vi "Koheras_AOTF.vi"(10 "String":string, 11 "VISA resource name 2":refnum<visa-resource-name>) -> (0 "error out":errorcluster, 2 "read buffer":string)   [LabVIEW 2009]
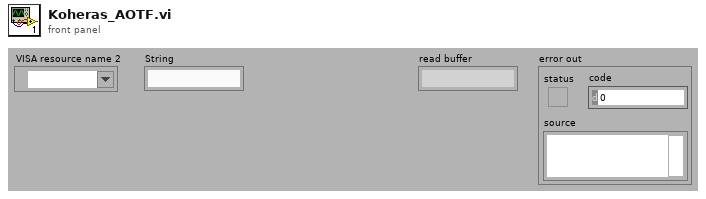
[diagram p1: front panel]
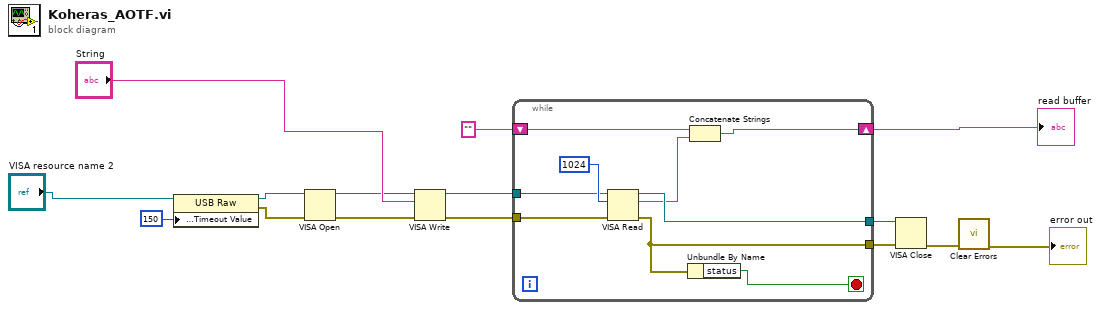
[diagram p0: block diagram]
diagram:
  n1 = property class="USB Raw"(reference="VISA resource name 2", "General Settings:Timeout Value"=u32 150) -> (reference out=w3:refnum<visa-resource-name>, error out=w2:errorcluster)  [unwired: 1 in]
  n2 = VISA Open(error in (no error)=w2, VISA resource name=w3) -> (VISA resource name=w8:refnum<visa-resource-name>, error out=w7:errorcluster)  [unwired: 3 out]
  n3 = VISA Write(VISA resource name=w8, write buffer="String", error in (no error)=w7) -> (VISA resource name out=w15:refnum<visa-resource-name>, error out=w14:errorcluster)  [unwired: 1 out]
  n4 = while {
    tunnel: w15 -> [w19]
    tunnel: w14 -> [w18]
    shift-right: [w21] -> w12
    shift-left: "" ("read buffer") -> [w24]
    tunnel: [w23] -> w10
    tunnel: [w17] -> w9
    stop <- w16 stop-if-true
    n5 = VISA Read(VISA resource name=w19, byte count=u32 1024, error in (no error)=w18) -> (VISA resource name out=w23:refnum<visa-resource-name>, read buffer=w20:string, error out=w17:errorcluster)  [unwired: 1 out]
    n6 = Unbundle By Name(w17) -> ("status"=w16:bool)
    n7 = Concatenate Strings(w24, w20) -> (w21:string)
  }
  "read buffer" <- w12
  n8 = VISA Close(VISA resource name=w10, error in (no error)=w9) -> (error out=w6:errorcluster)
  n9 = call <vilib>:"Clear Errors.vi"("error in (no error)"=w6) -> ("error out"=→"error out":errorcluster)  [unwired: 6 out]
